vi "Close shutter on error.vi"(8 "error in (no error)":errorcluster, 11 "Tomo in":refnum<class "Invivo_Tomo.lvclass">) -> (0 "error out":errorcluster, 3 "Tomo out":refnum<class "Invivo_Tomo.lvclass">)   [LabVIEW 2012, in "Invivo_Tomo.lvclass"]
uses:
  Invivo_Tomo.lvclass
  <vilib>/Distrio/Murmex/GenericMessage/GenericMessage.lvclass
  <vilib>/Distrio/Murmex/Message/Add or replace parameter.vi
  <vilib>/Distrio/Murmex/Murmex/Murmex.lvclass
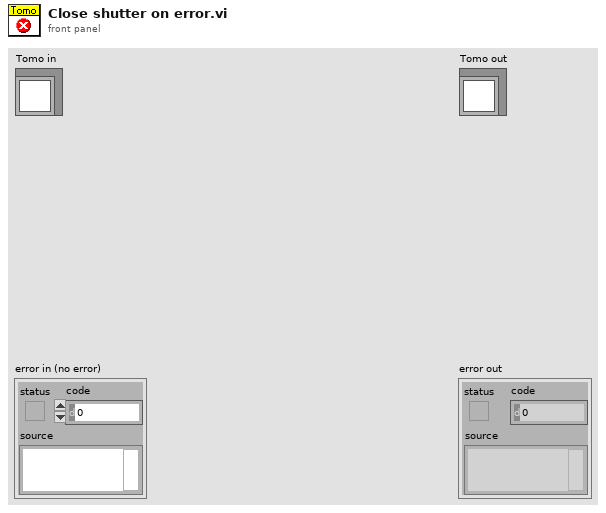
[diagram p1: front panel]
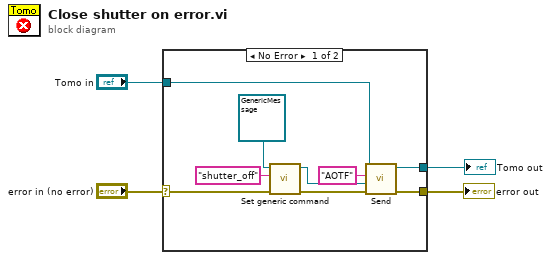
[diagram p0: block diagram]
diagram:
  n1 = case shown="No Error" "error in (no error)" {
    selector: "error in (no error)" -> [w11 w15]
    tunnel: [w10 w15] -> w3
    tunnel: [w5 w14] -> w1
    tunnel: "Tomo in" -> [w6 w14]
    frame No Error {
      n2 = call <vilib>:"Set generic command.vi"("error in (no error)"=w11, "generic command"="shutter_off", "GenericMessage in"=refnum<class "GenericMessage.lvclass"> refnum ("Distrio Murmex 1.1:GenericMessage")) -> ("error out"=w12:errorcluster, "GenericMessage out"=w8:refnum<class "GenericMessage.lvclass">)  [unwired: 7 in]
      n3 = call <vilib>:"Send.vi"("error in (no error)"=w12, "Message"=w8, "recipient"="AOTF", "Murmex in"=w6) -> ("error out"=w10:errorcluster, "Murmex out"=w5:refnum<class "Invivo_Tomo.lvclass">)  [unwired: 6 in]
    }
    frame Error {
    }
  }
  "error out" <- w3
  "Tomo out" <- w1
